vi "Local Transition.vi"(8 "error in (no error)":errorcluster, 10 "Target":refnum<class "State Machine.lvclass">, 11 "State Machine in":refnum<class "State Machine.lvclass">) -> (0 "error out":errorcluster, 2 "Nested State's Enqueuer":refnum<class "Message Enqueuer.lvclass">, 3 "State Machine out":refnum<class "State Machine.lvclass">)   [LabVIEW 2024]
uses:
  State Machine.lvclass
  <vilib>/ActorFramework/Message Enqueuer/Message Enqueuer.lvclass
  State Machine.lvclass/State Machine.ctl
  <vilib>/ActorFramework/Actor/Actor.lvclass
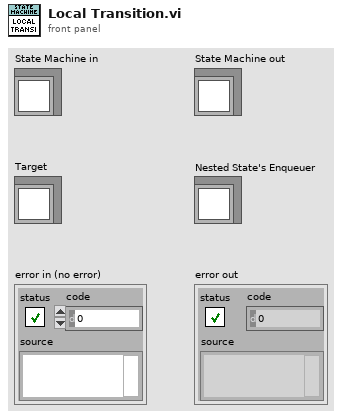
[diagram p1: front panel]
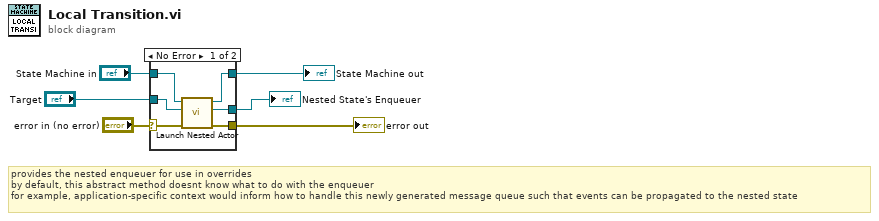
[diagram p0: block diagram]
diagram:
  # "provides the nested enqueuer for use in overrides\nby default, this abstract method doesnt know what to do with the enqueuer\nfor example, application-specific context would inform how to handle this newly generated message queue such that events can be propagated to the nested state"
  n1 = case shown="No Error" "error in (no error)" {
    selector: "error in (no error)" -> [w9 w14]
    tunnel: [w8 w14] -> w5
    tunnel: [w10 w13] -> w3
    tunnel: "State Machine in" -> [w11 w13]
    tunnel: "Target" -> [w12 _]
    tunnel: [w7 _] -> w1
    frame No Error {
      n2 = call <vilib>:"Launch Nested Actor.vi"("error in (no error)"=w9, "Nested Actor"=w12, "Caller Actor in"=w11) -> ("error out"=w8:errorcluster, "Nested Actor's Enqueuer"=w7:refnum<class "Message Enqueuer.lvclass">, "Caller Actor out"=w10:refnum<class "State Machine.lvclass">)  [unwired: 6 in]
    }
    frame Error {
    }
  }
  "error out" <- w5
  "State Machine out" <- w3
  "Nested State's Enqueuer" <- w1
